vi "Load App.vi"(8 "error in (no error)":cluster{"状态":bool, "代码":i32, "源":string} caption="错误输入（无错误）", 11 "状态通知器":refnum<notifier>) -> (0 "error out":cluster{"状态":bool, "代码":i32, "源":string} caption="错误输出")   [LabVIEW 2013, in "操作者框架.lvlib" / "操作者框架.lvclass"]
doc: "将应用程序加载至内存并使应用程序开始运行。输入通知器用于将文本发送至初始屏幕，以便向用户显示加载进程当前的状态。"
uses:
  <vilib>/ActorFramework/Message Queue/Message Queue.lvclass/Message Queue.ctl
  <vilib>/ActorFramework/Actor/Actor.lvclass
  <vilib>/ActorFramework/Message Queue/Message Queue.lvclass
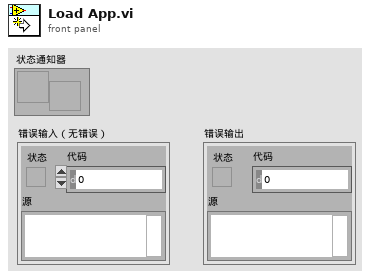
[diagram p1: front panel]
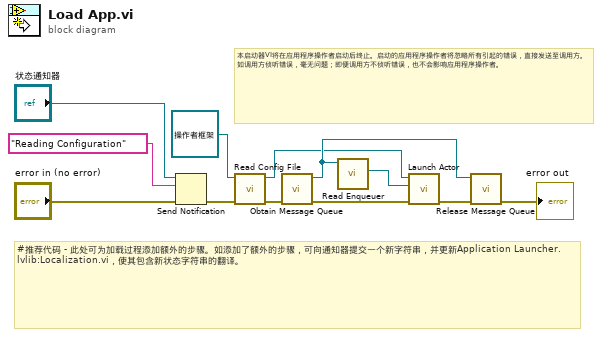
[diagram p0: block diagram]
diagram:
  # "本启动器VI将在应用程序操作者启动后终止。启动的应用程序操作者将忽略所有引起的错误，直接发送至调用方。如调用方侦听错误，毫无问题；即便调用方不侦听错误，也不会影响应用程序操作者。"
  # "#推荐代码 - 此处可为加载过程添加额外的步骤。如添加了额外的步骤，可向通知器提交一个新字符串，并更新Application Launcher.lvlib:Localization.vi，使其包含新状态字符串的翻译。"
  n1 = Send Notification(notification="Reading Configuration", notifier="状态通知器", error in (no error)="error in (no error)") -> (error out=w8:errorcluster)  [unwired: 1 out]
  n2 = call-dynamic "Read Config File.vi"("error in (no error)"=w8, "操作者框架输入"=refnum<class "操作者框架.lvclass"> refnum ("My Application.lvclass")) -> ("error out"=w4:cluster{"状态":bool, "代码":i32, "源":string}, "操作者框架输出"=w1:refnum<class "操作者框架.lvclass">)  [unwired: 8 in]
  n3 = call <vilib>:"Obtain Message Queue.vi"("error in (no error)"=w4) -> ("error out"=w3:errorcluster, "Message Queue"=w2:refnum<class "Message Queue.lvclass">)  [unwired: 9 in]
  n4 = call <vilib>:"Read Enqueuer.vi"("Message Queue"=w2) -> ("Message Enqueuer"=w7:refnum<class "Message Enqueuer.lvclass">)  [unwired: 10 in]
  n5 = call <vilib>:"Launch Actor.vi"("error in (no error)"=w3, "Actor-to-Caller Enqueuer"=w7, "Actor"=w1) -> ("error out"=w6:errorcluster)  [unwired: 7 in, 1 out]
  n6 = call <vilib>:"Release Message Queue.vi"("error in (no error)"=w6, "Message Queue"=w2) -> ("error out"=→"error out":errorcluster)  [unwired: 8 in, 1 out]
